vi "仪器全部断电.vi"   [LabVIEW 2016]
uses:
  PLC/PLC.lvlib
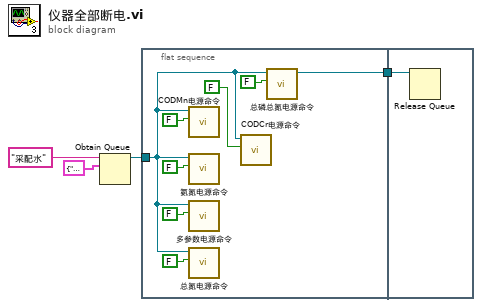
[diagram p0: block diagram]
diagram:
  n1 = Obtain Queue(name (unnamed)="采配水" ("名称（未命名）"), element data type=cluster{"命令":string, "数据":variant} {"命令"="", "数据"=variant}) -> (queue out=w2:refnum<queue>)  [unwired: 3 in, 2 out]
  n2 = flat-sequence {
    tunnel: w2 -> [w6]
    tunnel: [w5] -> w1
    tunnel: w1 -> [w13]
    frame #0 {
      n3 = call "CODMn电源命令.vi"("通电/断电"=FALSE, "队列"=w6) -> ()  [unwired: 9 in, 1 out]
      n4 = call "氨氮电源命令.vi"("通电/断电"=FALSE, "队列"=w6) -> ()  [unwired: 9 in, 1 out]
      n5 = call "多参数电源命令.vi"("通电/断电"=FALSE, "队列"=w6) -> ()  [unwired: 9 in, 1 out]
      n6 = call "总氮电源命令.vi"("通电/断电"=FALSE, "队列"=w6) -> ()  [unwired: 9 in, 1 out]
      n7 = call "CODCr电源命令.vi"("通电/断电"=FALSE, "队列"=w6) -> ()  [unwired: 9 in, 1 out]
      n8 = call "总磷总氮电源命令.vi"("通电/断电"=FALSE, "队列"=w6) -> ("队列输出"=w5:refnum<queue>)  [unwired: 9 in]
    }
    frame #1 {
      n9 = Release Queue(queue=w13) -> ()  [unwired: 2 in, 3 out]
    }
  }
